vi "DSF.Engine.Memory.Cache.Plugin.Get Transfer Group Caches.vi"(11 "Plugin Cache in":refnum<class "DSF.Engine.Memory.Cache.Plugin.lvclass">) -> (2 "Transfer Group Caches":refnum<class "DSF.Engine.Memory.Cache.Transfer Group.lvclass">[](array[class]), 3 "Plugin Cache out":refnum<class "DSF.Engine.Memory.Cache.Plugin.lvclass">)   [LabVIEW 2017, in "DSF.Engine.lvlib" / "DSF.Engine.Memory.Cache.Plugin.lvclass"]
uses:
  DSF.Engine.Memory.Cache.Plugin.lvclass
  DSF.Engine.Memory.Cache.Transfer Group.lvclass
  DSF.Engine.Memory.Cache.Plugin.lvclass/DSF.Engine.Memory.Cache.Plugin.ctl
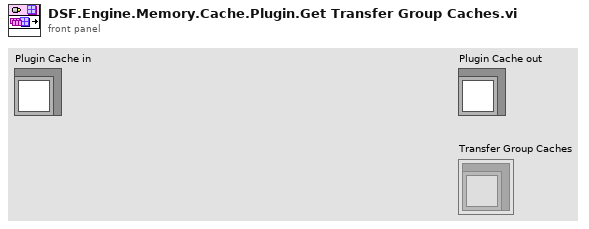
[diagram p1: front panel]
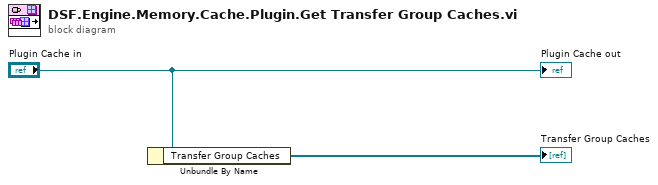
[diagram p0: block diagram]
diagram:
  n1 = Unbundle By Name("Plugin Cache in") -> ("Transfer Group Caches"=→"Transfer Group Caches":refnum<class "DSF.Engine.Memory.Cache.Transfer Group.lvclass">[])
  "Plugin Cache out" <- "Plugin Cache in"
